vi "RegionData.vi"(0 "Action":u32(ring) items=["Reset", "Read Array", "Read Element", "Write Element", "Write Array"], 1 "Array No.":i32, 2 "Array Size / Index":i32, 3 "Data IN":dbl format="%.2f", 4 "Array IN":dbl[](array[numeric]) format="%.2f") -> (5 "Data OUT":dbl format="%.2f", 6 "Array OUT":dbl[](array[numeric]) format="%.2f")   [LabVIEW 2013]
doc: "Reset data arrays, or read/write array elements, or read entire\narrays.\nAction: 0 Reset arrays\n 1 Read array\n 2 Read array element\n 3 Write array element"
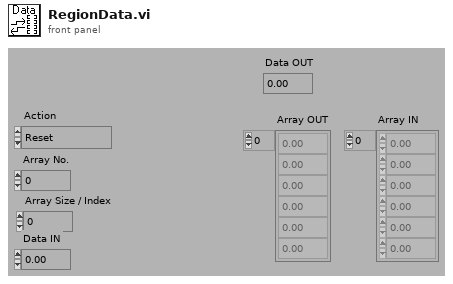
[diagram p1: front panel]
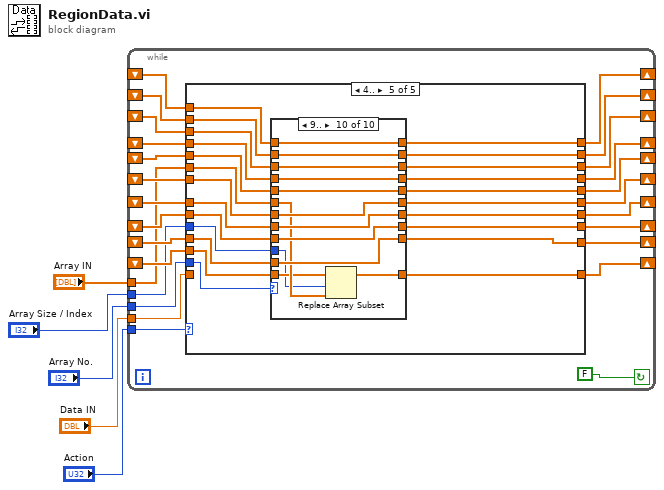
[diagram p0: block diagram]
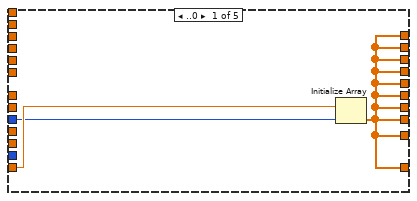
[diagram p2: hidden frame]
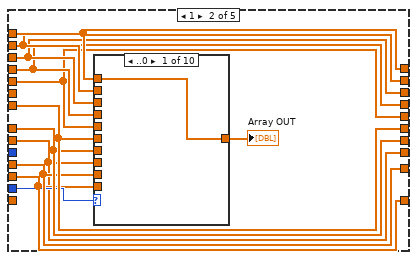
[diagram p3: hidden frame]
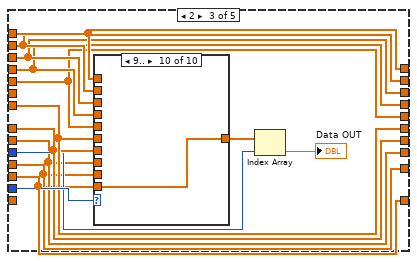
[diagram p13: hidden frame]
diagram:
  n1 = while {
    shift-left: _ -> [w11]
    shift-right: [w10] -> _
    tunnel: "Array No." -> [w12]
    shift-left: _ -> [w13]
    shift-right: [w21] -> _
    shift-left: _ -> [w14]
    shift-right: [w9] -> _
    shift-left: _ -> [w15]
    shift-right: [w22] -> _
    shift-left: _ -> [w16]
    shift-right: [w23] -> _
    shift-left: _ -> [w17]
    shift-right: [w24] -> _
    shift-left: _ -> [w18]
    shift-right: [w25] -> _
    shift-left: _ -> [w19]
    shift-right: [w26] -> _
    shift-left: _ -> [w20]
    shift-right: [w27] -> _
    tunnel: "Data IN" -> [w29]
    tunnel: "Array Size / Index" -> [w7]
    tunnel: "Action" -> [w31]
    shift-left: _ -> [w30]
    shift-right: [w28] -> _
    tunnel: "Array IN" -> [w6]
    stop <- FALSE continue-if-true
    n2 = case shown="4.." w31 {
      tunnel: [w34 w46 w69 w99 w245] -> w28
      tunnel: w30 -> [_ w46 w69 w103 w256]
      tunnel: w7 -> [w32 _ w61 w100 w254]
      tunnel: w29 -> [w33 _ _ w101 _]
      tunnel: [w34 w44 w67 w90 w244] -> w27
      tunnel: [w34 w43 w66 w89 w243] -> w26
      tunnel: [w34 w42 w65 w88 w242] -> w25
      tunnel: [w34 w41 w64 w85 w241] -> w24
      tunnel: [w34 w40 w63 w83 w240] -> w23
      tunnel: [w34 w39 w62 w87 w239] -> w22
      tunnel: [w34 w35 w59 w81 w238] -> w9
      tunnel: [w34 w38 w58 w82 w237] -> w21
      tunnel: w20 -> [_ w44 w67 w98 w255]
      tunnel: w19 -> [_ w43 w66 w97 w253]
      tunnel: w18 -> [_ w42 w65 w96 w252]
      tunnel: w17 -> [_ w41 w64 w95 w251]
      tunnel: w16 -> [_ w40 w63 w84 w250]
      tunnel: w15 -> [_ w39 w62 w94 w249]
      tunnel: w14 -> [_ w35 w59 w93 w248]
      tunnel: w13 -> [_ w38 w58 w92 w247]
      tunnel: w12 -> [_ w37 w70 w102 w235]
      tunnel: w11 -> [_ w36 w57 w91 w246]
      tunnel: [w34 w36 w57 w86 w236] -> w10
      tunnel: w6 -> [_ _ _ _ w234]
      frame ..0 {
        n3 = Initialize Array(w33, w32) -> (w34:dbl[])
      }
      frame 1 {
        n4 = case shown="..0" w37 {
          tunnel: w46 -> [w47 _ _ _ _ _ _ _ _ _]
          tunnel: [w47 w48 w49 w50 w51 w52 w53 w54 w55 w56] -> w45
          tunnel: w44 -> [_ w48 _ _ _ _ _ _ _ _]
          tunnel: w43 -> [_ _ w49 _ _ _ _ _ _ _]
          tunnel: w42 -> [_ _ _ w50 _ _ _ _ _ _]
          tunnel: w41 -> [_ _ _ _ w51 _ _ _ _ _]
          tunnel: w40 -> [_ _ _ _ _ w52 _ _ _ _]
          tunnel: w39 -> [_ _ _ _ _ _ w53 _ _ _]
          tunnel: w35 -> [_ _ _ _ _ _ _ w54 _ _]
          tunnel: w38 -> [_ _ _ _ _ _ _ _ w55 _]
          tunnel: w36 -> [_ _ _ _ _ _ _ _ _ w56]
          frame ..0 {
          }
          frame 1 {
          }
          frame 2 {
          }
          frame 3 {
          }
          frame 4 {
          }
          frame 5 {
          }
          frame 6 {
          }
          frame 7 {
          }
          frame 8 {
          }
          frame 9.. {
          }
        }
        "Array OUT" <- w45
      }
      frame 2 {
        n5 = case shown="9.." w70 {
          tunnel: w69 -> [w71 _ _ _ _ _ _ _ _ _]
          tunnel: [w71 w72 w73 w74 w75 w76 w77 w78 w79 w80] -> w68
          tunnel: w67 -> [_ w72 _ _ _ _ _ _ _ _]
          tunnel: w66 -> [_ _ w73 _ _ _ _ _ _ _]
          tunnel: w65 -> [_ _ _ w74 _ _ _ _ _ _]
          tunnel: w64 -> [_ _ _ _ w75 _ _ _ _ _]
          tunnel: w63 -> [_ _ _ _ _ w76 _ _ _ _]
          tunnel: w62 -> [_ _ _ _ _ _ w77 _ _ _]
          tunnel: w59 -> [_ _ _ _ _ _ _ w78 _ _]
          tunnel: w58 -> [_ _ _ _ _ _ _ _ w79 _]
          tunnel: w57 -> [_ _ _ _ _ _ _ _ _ w80]
          frame ..0 {
          }
          frame 1 {
          }
          frame 2 {
          }
          frame 3 {
          }
          frame 4 {
          }
          frame 5 {
          }
          frame 6 {
          }
          frame 7 {
          }
          frame 8 {
          }
          frame 9.. {
          }
        }
        n6 = Index Array(array=w68, index=w61) -> (element=→"Data OUT":dbl)
      }
      frame 3 {
        n7 = case shown="9.." w102 {
          tunnel: w103 -> [w114 w129 w142 w155 w168 w181 w194 w207 w220 w233]
          tunnel: w101 -> [w116 w128 w138 w150 w162 w174 w186 w198 w211 w224]
          tunnel: w100 -> [w115 w127 w137 w149 w161 w173 w185 w197 w210 w221]
          tunnel: [w113 w129 w142 w155 w168 w181 w194 w207 w220 w233] -> w99
          tunnel: w98 -> [w111 w126 w141 w154 w167 w180 w193 w206 w219 w232]
          tunnel: w97 -> [w110 w124 w140 w153 w166 w179 w192 w205 w218 w231]
          tunnel: w96 -> [w109 w123 w136 w152 w165 w178 w191 w204 w217 w230]
          tunnel: w95 -> [w108 w122 w135 w148 w164 w177 w190 w203 w216 w229]
          tunnel: w94 -> [w107 w120 w133 w146 w159 w172 w188 w201 w214 w227]
          tunnel: w93 -> [w106 w119 w132 w145 w158 w171 w184 w200 w213 w226]
          tunnel: w92 -> [w105 w118 w131 w144 w157 w170 w183 w196 w212 w225]
          tunnel: w91 -> [w104 w117 w130 w143 w156 w169 w182 w195 w208 w223]
          tunnel: [w106 w119 w132 w145 w158 w171 w184 w199 w213 w226] -> w81
          tunnel: [w104 w117 w130 w143 w156 w169 w182 w195 w208 w222] -> w86
          tunnel: [w112 w121 w134 w147 w160 w175 w189 w202 w215 w228] -> w83
          tunnel: w84 -> [w112 w121 w134 w147 w160 w176 w189 w202 w215 w228]
          tunnel: [w109 w123 w136 w151 w165 w178 w191 w204 w217 w230] -> w88
          tunnel: [w105 w118 w131 w144 w157 w170 w183 w196 w209 w225] -> w82
          tunnel: [w111 w125 w141 w154 w167 w180 w193 w206 w219 w232] -> w90
          tunnel: [w110 w124 w139 w153 w166 w179 w192 w205 w218 w231] -> w89
          tunnel: [w108 w122 w135 w148 w163 w177 w190 w203 w216 w229] -> w85
          tunnel: [w107 w120 w133 w146 w159 w172 w187 w201 w214 w227] -> w87
          frame ..0 {
            n8 = Replace Array Subset(array=w114, new element=w116, index=w115) -> (w113:dbl[])
          }
          frame 1 {
            n9 = Replace Array Subset(array=w126, new element=w128, index=w127) -> (w125:dbl[])
          }
          frame 2 {
            n10 = Replace Array Subset(array=w140, new element=w138, index=w137) -> (w139:dbl[])
          }
          frame 3 {
            n11 = Replace Array Subset(array=w152, new element=w150, index=w149) -> (w151:dbl[])
          }
          frame 4 {
            n12 = Replace Array Subset(array=w164, new element=w162, index=w161) -> (w163:dbl[])
          }
          frame 5 {
            n13 = Replace Array Subset(array=w176, new element=w174, index=w173) -> (w175:dbl[])
          }
          frame 6 {
            n14 = Replace Array Subset(array=w188, new element=w186, index=w185) -> (w187:dbl[])
          }
          frame 7 {
            n15 = Replace Array Subset(array=w200, new element=w198, index=w197) -> (w199:dbl[])
          }
          frame 8 {
            n16 = Replace Array Subset(array=w212, new element=w211, index=w210) -> (w209:dbl[])
          }
          frame 9.. {
            n17 = Replace Array Subset(array=w223, new element=w224, index=w221) -> (w222:dbl[])
          }
        }
      }
      frame 4.. {
        n18 = case shown="9.." w235 {
          tunnel: w256 -> [w267 w282 w295 w308 w321 w334 w347 w360 w373 w386]
          tunnel: w234 -> [w269 w281 w291 w303 w315 w327 w339 w351 w364 w377]
          tunnel: w254 -> [w268 w280 w290 w302 w314 w326 w338 w350 w363 w374]
          tunnel: [w266 w282 w295 w308 w321 w334 w347 w360 w373 w386] -> w245
          tunnel: w255 -> [w264 w279 w294 w307 w320 w333 w346 w359 w372 w385]
          tunnel: w253 -> [w263 w277 w293 w306 w319 w332 w345 w358 w371 w384]
          tunnel: w252 -> [w262 w276 w289 w305 w318 w331 w344 w357 w370 w383]
          tunnel: w251 -> [w261 w275 w288 w301 w317 w330 w343 w356 w369 w382]
          tunnel: w249 -> [w260 w273 w286 w299 w312 w325 w341 w354 w367 w380]
          tunnel: w248 -> [w259 w272 w285 w298 w311 w324 w337 w353 w366 w379]
          tunnel: w247 -> [w258 w271 w284 w297 w310 w323 w336 w349 w365 w378]
          tunnel: w246 -> [w257 w270 w283 w296 w309 w322 w335 w348 w361 w376]
          tunnel: [w259 w272 w285 w298 w311 w324 w337 w352 w366 w379] -> w238
          tunnel: [w257 w270 w283 w296 w309 w322 w335 w348 w361 w375] -> w236
          tunnel: [w265 w274 w287 w300 w313 w328 w342 w355 w368 w381] -> w240
          tunnel: w250 -> [w265 w274 w287 w300 w313 w329 w342 w355 w368 w381]
          tunnel: [w262 w276 w289 w304 w318 w331 w344 w357 w370 w383] -> w242
          tunnel: [w258 w271 w284 w297 w310 w323 w336 w349 w362 w378] -> w237
          tunnel: [w264 w278 w294 w307 w320 w333 w346 w359 w372 w385] -> w244
          tunnel: [w263 w277 w292 w306 w319 w332 w345 w358 w371 w384] -> w243
          tunnel: [w261 w275 w288 w301 w316 w330 w343 w356 w369 w382] -> w241
          tunnel: [w260 w273 w286 w299 w312 w325 w340 w354 w367 w380] -> w239
          frame ..0 {
            n19 = Replace Array Subset(array=w267, new element=w269, index=w268) -> (w266:dbl[])
          }
          frame 1 {
            n20 = Replace Array Subset(array=w279, new element=w281, index=w280) -> (w278:dbl[])
          }
          frame 2 {
            n21 = Replace Array Subset(array=w293, new element=w291, index=w290) -> (w292:dbl[])
          }
          frame 3 {
            n22 = Replace Array Subset(array=w305, new element=w303, index=w302) -> (w304:dbl[])
          }
          frame 4 {
            n23 = Replace Array Subset(array=w317, new element=w315, index=w314) -> (w316:dbl[])
          }
          frame 5 {
            n24 = Replace Array Subset(array=w329, new element=w327, index=w326) -> (w328:dbl[])
          }
          frame 6 {
            n25 = Replace Array Subset(array=w341, new element=w339, index=w338) -> (w340:dbl[])
          }
          frame 7 {
            n26 = Replace Array Subset(array=w353, new element=w351, index=w350) -> (w352:dbl[])
          }
          frame 8 {
            n27 = Replace Array Subset(array=w365, new element=w364, index=w363) -> (w362:dbl[])
          }
          frame 9.. {
            n28 = Replace Array Subset(array=w376, new element=w377, index=w374) -> (w375:dbl[])
          }
        }
      }
    }
  }
